vi "Test2.vi"() -> ()   [LabVIEW 2011]
panel:
  in  "Boolean 9":bool
  in  "Boolean 8":bool
  in  "Boolean 7":bool
  in  "Boolean 6":bool
  in  "Boolean 5":bool
  out "Boolean 4":bool
  in  "Boolean 3":bool
  in  "Boolean 2":bool
  in  "OK Button":bool
  in  "Boolean":bool
  in  "Test":bool
  in  "Blank":bool
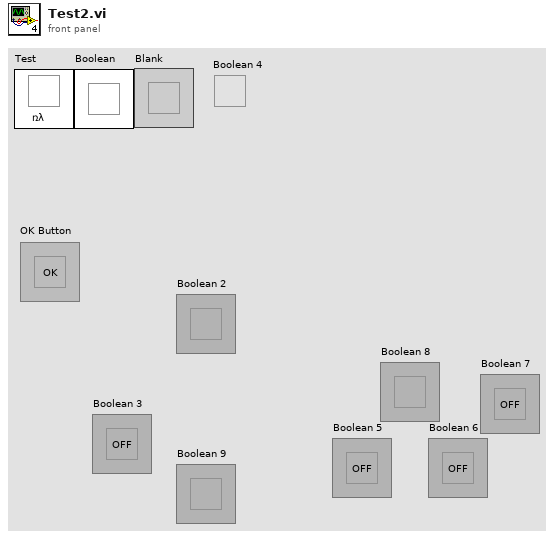
[diagram p1: front panel]
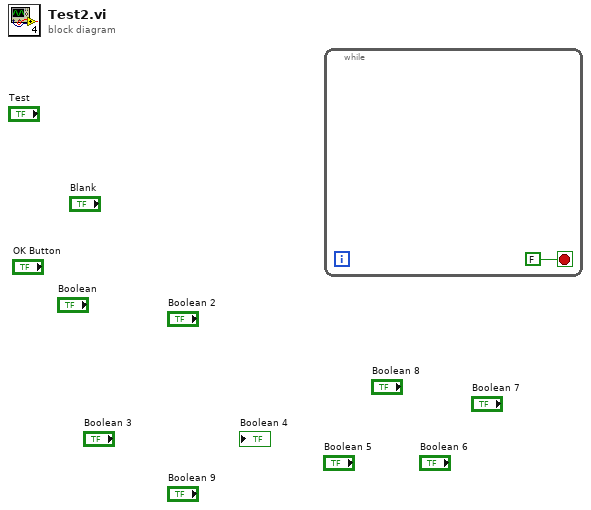
[diagram p0: block diagram]
diagram:
  n1 = while {
    stop <- FALSE stop-if-true
  }
